vi "storage_RectCentroid_copy.vi"(1 "rect":T1) -> (0 "point":cluster{"x":i16, "y":i16})   [LabVIEW 2017]
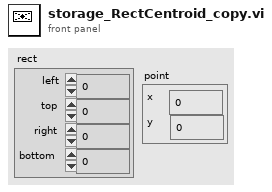
[diagram p1: front panel]
types:
  T1 = cluster{"left":i16, "top":i16, "right":i16, "bottom":i16}
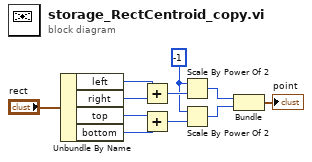
[diagram p0: block diagram]
diagram:
  w4 = -1
  n1 = Unbundle By Name("rect") -> ("left"=w10:i16, "right"=w9:i16, "top"=w8:i16, "bottom"=w7:i16)
  n2 = Add(x=w10, y=w9) -> (x+y=w5:i16)
  n3 = Add(x=w8, y=w7) -> (x+y=w6:i16)
  n4 = Scale By Power Of 2(n=w4, x=w5) -> (x*2^n=w3:i16)
  n5 = Scale By Power Of 2(n=w4, x=w6) -> (x*2^n=w2:i16)
  n6 = Bundle(w3, w2) -> (→"point":cluster{i16, i16})  [unwired: 1 in]
